vi "Supported Devices.vi"() -> (3 "Supported Devices":string[](array[string]))   [LabVIEW 2025, in "I2C Bus Monitor UI.lvlib"]
uses:
  I2C Bus Monitor UI.lvlib
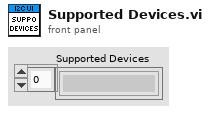
[diagram p1: front panel]
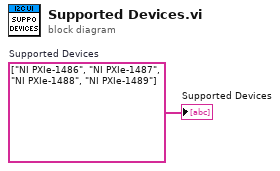
[diagram p0: block diagram]
diagram:
  w1 = string[] ["NI PXIe-1486", "NI PXIe-1487", "NI PXIe-1488", "NI PXIe-1489"]  # Supported Devices
  "Supported Devices" <- w1
